vi "test_libssh2_channel_get_exit_signal.vi"() -> ()   [LabVIEW 2013, in "libssh2_integration_tests.lvlib"]
uses:
  libssh2_integration_tests.lvlib
  <vilib>/addons/_JKI Toolkits/Caraya/classes/Test/Test.lvclass
  libssh2/libssh2.lvlib
  <vilib>/addons/_JKI Toolkits/Caraya/classes/Assert/Assert.lvclass
panel:
  out "error out":errorcluster
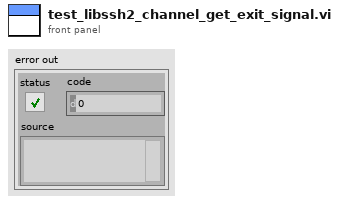
[diagram p1: front panel]
types:
  T1 = typedef "libssh2.lvlib/Session Refnum.ctl" = refnum<k1>
  T2 = typedef "libssh2.lvlib/Channel Refnum.ctl" = refnum<k1>
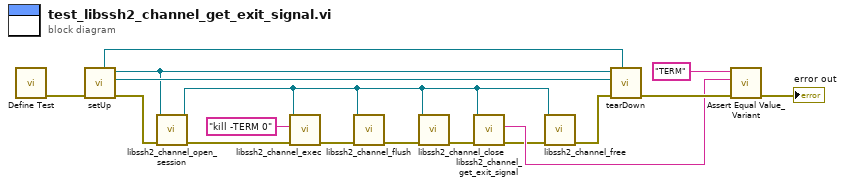
[diagram p0: block diagram]
diagram:
  n1 = call <vilib>:"Define Test.vi"() -> ("error out"=w16:errorcluster)  [unwired: 10 in, 1 out]
  n2 = call "setUp.vi"("error in (no error)"=w16) -> ("error out"=w13:errorcluster, "connection ID"=w8:refnum<k5>, "session"=w7:T1, "fixture"=w14:refnum<class "Server Fixture.lvclass">)  [unwired: 7 in]
  n3 = call "libssh2_channel_open_session.vi"("error in (no error)"=w13, "session"=w7) -> ("error out"=w4:errorcluster, "channel"=w1:T2)  [unwired: 8 in]
  n4 = call "libssh2_channel_exec.vi"("error in (no error)"=w4, "command"="kill -TERM 0", "channel"=w1) -> ("error out"=w3:errorcluster)  [unwired: 8 in]
  n5 = call "libssh2_channel_flush.vi"("error in (no error)"=w3, "channel"=w1) -> ("error out"=w2:errorcluster)  [unwired: 9 in]
  n6 = call "libssh2_channel_close.vi"("error in (no error)"=w2, "channel"=w1) -> ("error out"=w6:errorcluster)  [unwired: 9 in]
  n7 = call "libssh2_channel_get_exit_signal.vi"("error in (no error)"=w6, "channel"=w1) -> ("error out"=w9:errorcluster, "exitsignal"=w11:string)  [unwired: 6 in, 2 out]
  n8 = call "libssh2_channel_free.vi"("error in (no error)"=w9, "channel"=w1) -> ("error out"=w12:errorcluster)  [unwired: 9 in]
  n9 = call "tearDown.vi"("fixture"=w14, "error in (no error)"=w12, "connection ID"=w8, "session"=w7) -> ("error out"=w15:errorcluster)  [unwired: 7 in]
  n10 = call <vilib>:"Assert Equal Value_Variant.vi"("error in (no error)"=w15, "Y"=w11, "X"="TERM" ("exitsignal")) -> ("error out"=→"error out":errorcluster)  [unwired: 7 in, 1 out]
